vi "ni5660 Sub 562x Ready.vi"(0 "instrument handle in":refnum<k15>, 7 "PLL lock time (sec)":dbl=1.0 min=0.0 format="%.2f", 9 "max timeout (sec)":dbl=6.0 min=0.0 format="%.2f", 11 "error in (no error)":errorcluster) -> (4 "instrument handle out":refnum<k15>, 15 "error out":errorcluster)   [LabVIEW 2011]
doc: "This VI will wait until the phase-locked loop (PLL) of the NI 5620 has been locked to the 10 MHz reference clock for a minimum amount of time (PLL lock time) or until its timeout expires, whichever happens first. It will return an error if a timeout occurs.\n\nSetting the PLL lock time to 0 seconds causes this VI to not wait for the PLL to settle before returning, and prevents the timeout error from occurring.\n\nThe first time the NI 5620 locks to a reference clock source, it can take up to about five seconds. However, if the reference clock source (e.g. front connector, PXI backplane clock) is not changed, the time needed to lock reduces to one second. The 'PLL lock time' control has a default value of one second, but you should increase this value to four seconds (recommended value) for applications involving phase measurements. This is due to the fact that the 'PLL Locked' property node returns a TRUE value before the PLL has finished settling to a level suitable for making phase measurements. For highest accuracy, you should make phase measurements after the PLL has settled, and empirical tests show that the PLL settles completely after four seconds."
panel:
  # "Minimum recommended PLL lock times:\n1 second for most measurements (default)\n4 seconds for phase measurements"
  # "Recommended max timeout value:\nPLL lock time + 5 seconds"
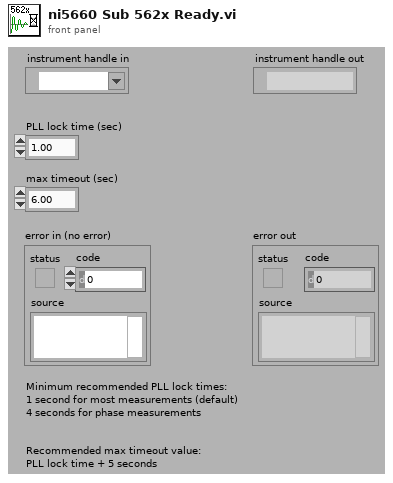
[diagram p1: front panel]
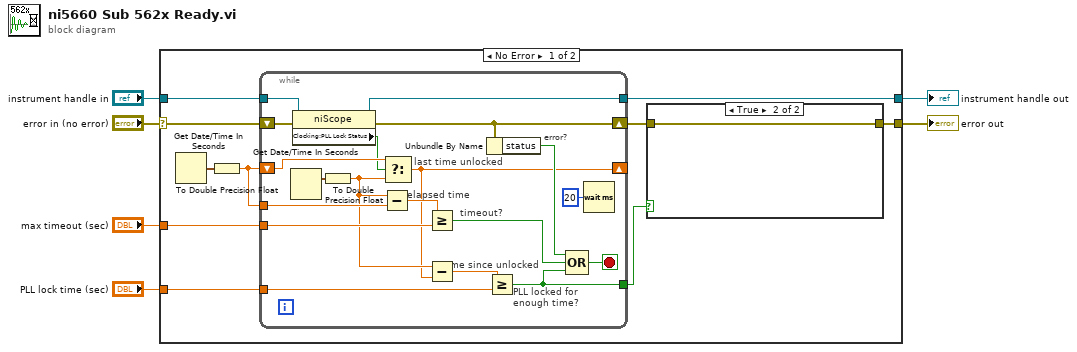
[diagram p0: block diagram]
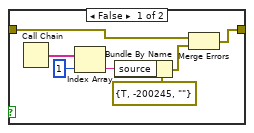
[diagram p2: hidden frame]
diagram:
  n1 = case shown="No Error" "error in (no error)" {
    selector: "error in (no error)" -> [w16 w45]
    tunnel: [w11 w44] -> w6
    tunnel: [w9 w45] -> w4
    tunnel: "instrument handle in" -> [w12 w44]
    tunnel: "max timeout (sec)" -> [w7 _]
    tunnel: "PLL lock time (sec)" -> [w13 _]
    frame No Error {
      n2 = Get Date/Time In Seconds() -> (seconds since 1Jan1904=w14:timestamp)
      n3 = To Double Precision Float(number=w14) -> (double precision float=w15:dbl)
      n4 = while {
        shift-right: [w18] -> _
        shift-left: w15 -> [w31]
        tunnel: w15 -> [w34]
        tunnel: w13 -> [w29]
        tunnel: w7 -> [w28]
        shift-right: [w23] -> w10
        shift-left: w16 -> [w24]
        tunnel: w12 -> [w21]
        tunnel: [w20] -> w11
        tunnel: [w19] -> w8
        stop <- w32 stop-if-true
        # "last time unlocked"
        # "error?"
        # "PLL locked for\nenough time?"
        # "timeout?"
        # "time since unlocked"
        # "elapsed time"
        n5 = Get Date/Time In Seconds() -> (seconds since 1Jan1904=w22:timestamp)
        n6 = property class="niScope"(reference=w21, error in=w24) -> (reference out=w20:refnum<k15>, error out=w23:errorcluster, "Clocking:PLL Lock Status"=w25:bool)
        n7 = To Double Precision Float(number=w22) -> (double precision float=w27:dbl)
        n8 = Subtract(x=w27, y=w34) -> (x-y=w33:dbl)
        n9 = Select(t=w31, s=w25, f=w27) -> (s? t:f=w18:dbl)
        n10 = Greater Or Equal?(x=w33, y=w28) -> (x >= y?=w17:bool)
        n11 = Subtract(x=w27, y=w18) -> (x-y=w35:dbl)
        n12 = Unbundle By Name(w23) -> ("status"=w30:bool)
        n13 = Greater Or Equal?(x=w35, y=w29) -> (x >= y?=w19:bool)
        n14 = Compound Arithmetic op=OR(w30, w17, w19) -> (w32:bool)
        n15 = Wait (ms)(milliseconds to wait=u32 20) -> ()  [unwired: 1 out]
      }
      n16 = case shown="True" w8 {
        tunnel: w10 -> [w41 w43]
        tunnel: [w39 w43] -> w9
        frame False {
          n17 = Call Chain() -> (call chain=w38:string[])
          n18 = Index Array(array=w38, index=1) -> (element=w36:string)
          n19 = Bundle By Name(cluster=errorcluster {"status"=TRUE, "code"=-200245, "source"=""} ("error in 2 (no error)"), "source"=w36) -> (w40:errorcluster)
          n20 = Merge Errors(w41, w40) -> (w39:errorcluster)
        }
        frame True {
        }
      }
    }
    frame Error {
    }
  }
  "instrument handle out" <- w6
  "error out" <- w4
